vi "tester.vi"() -> ()   [LabVIEW 2014]
panel:
  out "Current":i32
  in  "Desired":i32
  in  "stop":bool
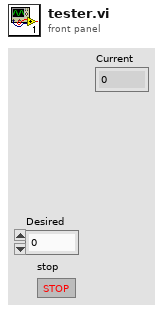
[diagram p1: front panel]
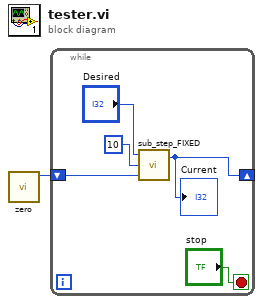
[diagram p0: block diagram]
diagram:
  n1 = call "zero.vi"() -> ("PositionOut"=w1:i32)  [unwired: 11 in]
  n2 = while {
    shift-right: [w2] -> _
    shift-left: w1 -> [w3]
    stop <- "stop" stop-if-true
    n3 = call "sub_step_FIXED.vi"("Current Position"=w3, "millisecond multiple"=u32 10, "Desired Position"="Desired") -> ("Position Out"=w2:i32)  [unwired: 1 in]
    "Current" <- w2
  }
